vi "CRYSet Tool Window.vi"(7 "VI Ref In":refnum<vi>, 8 "Height":i32, 9 "Width":i32, 10 "Top":i32, 11 "Left":i32) -> (3 "VI Ref Out":refnum<vi>)   [LabVIEW 2013]
uses:
  user32.dll
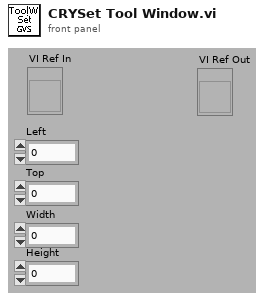
[diagram p1: front panel]
types:
  T1 = typedef "CRYWindow Refnum Strict Type Def.ctl" = refnum<k1>
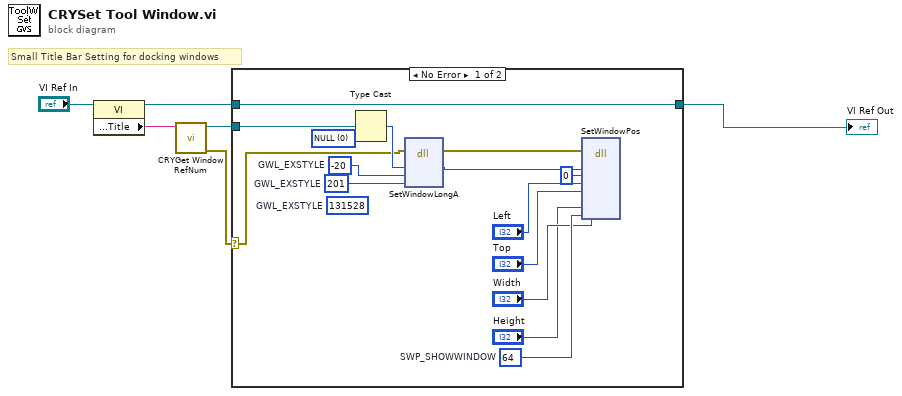
[diagram p0: block diagram]
diagram:
  # "Small Title Bar Setting for docking windows"
  n1 = property class="VI"(reference="VI Ref In") -> (reference out=w1:refnum<vi>, "Front Panel.Title"=w3:string)  [unwired: 1 in, 1 out]
  n2 = call "CRYGet Window RefNum.vi"("window name (\"\")"=w3) -> ("error out"=w4:errorcluster, "window refnum (NaWR)"=w6:T1)  [unwired: 1 in, 6 out]
  n3 = case shown="No Error" w4 {
    selector: w4 -> [w11 _]
    tunnel: w6 -> [w21 _]
    tunnel: w1 -> [w9 w22]
    tunnel: [w9 w22] -> w2
    frame No Error {
      (unwired) 131528  # GWL_EXSTYLE
      w7 = 201  # GWL_EXSTYLE
      w14 = u32 0 items=["NULL"]
      w13 = -20  # GWL_EXSTYLE
      w19 = 64  # SWP_SHOWWINDOW
      n4 = Type Cast(type=w14, x=w21) -> (*(type *) &x=w12:u32)
      n5 = dll-call lib="user32.dll" fn="SetWindowLongA"(error in=w11, "hWnd"=w12, "index"=w13, "dWNewLong"=w7) -> (error out=w10:errorcluster, "hWnd"=w20:u32)  [unwired: 4 in, 2 out]
      n6 = dll-call lib="user32.dll" fn="SetWindowPos"(error in=w10, "hWnd"=w20, "hWndInsertAfter"=u32 0, "left"="Left", "top"="Top", "width"="Width", "height"="Height", "fuFlags"=w19) -> ()  [unwired: 9 in, 3 out]
    }
    frame Error {
    }
  }
  "VI Ref Out" <- w2
